vi "LSMcontroller_v57.vi"() -> ()   [LabVIEW 2015] (continued)
                    n5196 = local write "Build digital waveform tabs"(w2028) -> ()
                    n5197 = local write "Digital DC (%)"(w2038) -> ()
                    n5198 = local write "Matlab waveform path DO"(w2029) -> ()
                    n5199 = local write "Sampling rate \ncurrent wf"(w2035) -> ()
                    n5200 = local write "Digital time offset (s)"(w2031) -> ()
                    n5201 = local write "Matlab padding value DO"(w2030) -> ()
                    n5202 = local write "Digital padding value"(w2030) -> ()
                    n5203 = local write "Digital Freq (Hz)"(w2036) -> ()
                    n5204 = local write "Digital phase (s)"(w2037) -> ()
                  }
                  frame True {
                  }
                }
              }
              frame #6 {
                n5205 = local read "finite samples"() -> (w2041:bool)
                n5206 = local read "continuous"() -> (w2042:bool)
                n5207 = local read "wavdet"() -> (w2043:bool)
                n5208 = call "2pparameters.vi"("command"="get") -> ("params out"=w2046:T12)  [unwired: 1 in]
                n5209 = Bundle By Name(cluster=w2046, "finite"=w2041, "cont"=w2042, "wavdet"=w2043) -> (w2044:T12)
                n5210 = call "2pparameters.vi"("Params in"=w2044, "command"="set") -> ()  [unwired: 1 out]
              }
            }
          }
          event "Exit": Value Change {
            n5211 = event-data() -> ("NewVal"=w2048:bool)  [unwired: 1 in]
          }
        }
        n5212 = Wait (ms)(milliseconds to wait=u32 50) -> ()  [unwired: 1 out]
      }
    }
    frame #3 {
      w6705 = FALSE ("Value (Signaling)")
      n5213 = property on="Start" class="Bool (strict)"("Val(Sgnl)"=w6705) -> ()  [unwired: 2 in, 2 out]
      n5214 = property on="Exit" class="Bool (strict)"("Val(Sgnl)"=w6705) -> ()  [unwired: 2 in, 2 out]
      n5215 = property on="Stop" class="Bool (strict)"("Val(Sgnl)"=w6705) -> ()  [unwired: 2 in, 2 out]
      n5216 = flat-sequence {
        frame #0 {
          w6706 = u16 1 items=["OD 0"=1, "OD 0.5"=2, "OD 1"=3, "OD 2"=4, "OD 3"=5, "OD 4"=6] ("New ODfilt")
          n5217 = local read "ODfilt"() -> (w6707:u16)
          n5218 = call "filterwheelcontrol_nothorlabslib.vi"("Current OD filt"=w6707, "New ODfilt"=w6706) -> ()  [unwired: 1 in]
        }
        frame #1 {
          n5219 = Wait (ms)(milliseconds to wait=u32 1000) -> ()  [unwired: 1 out]
        }
      }
    }
  }
